vi "Get Control Data.vi"(6 "offset":i32, 8 "error in (no error)":errorcluster, 11 "bitfile xml in":string) -> (0 "error out":errorcluster, 2 "Controls":T1[](array[typedef]), 3 "Indicators":T1[](array[typedef]), 4 "offset past EndTag":i32)   [LabVIEW 2010, in "FPGA Bitfile Utility.lvlib"]
uses:
  <userlib>/_FPGA Interface Advanced Tools/FPGA Bitfile Utility/FPGA Bitfile Utility.lvlib
  <userlib>/_FPGA Interface Advanced Tools/FPGA Bitfile Utility/TypeDefs/Control_Indicator Info.ctl
  <vilib>/rvi/DataTransferAndStorage/Container/Common/niFpgaDataTypeControl.ctl
  <vilib>/rvi/Utilities/XML/nirviXML_GetValue.vi
  <vilib>/rvi/Utilities/XML/nirviXML_GetValue_String.vi
  <vilib>/rvi/Bitfile/niFpgaReadBitfileXml_VIRegisterMap.vi
  <vilib>/rvi/Utilities/XML/nirviXML_GetValue_U32.vi
  <vilib>/Utility/VariantDataType/VariantType.lvlib
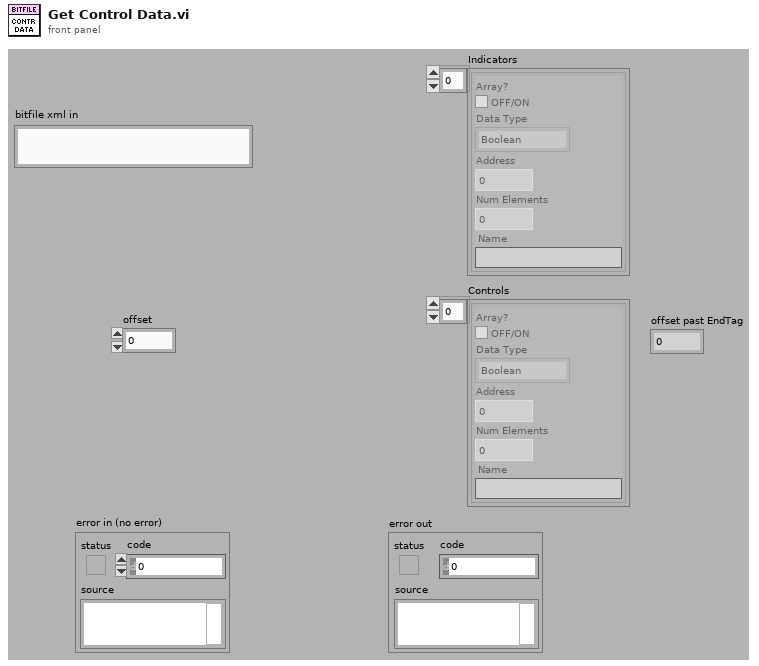
[diagram p1: front panel]
types:
  T1 = typedef "FPGA Bitfile Utility.lvlib/Control_Indicator Info.ctl" = cluster{"Array?":bool, "Data Type":T2, "Address":u32, "Num Elements":u32, "Name":string}
  T2 = typedef "niFpgaDataTypeControl.ctl" = enum32{"Boolean", "I8", "I16", "I32", "I64", "U8", "U16", "U32", "U64", "FXP", "CustomControl"}
  T3 = typedef "nirviControlStructure.ctl" = cluster{"Name":string, "Hidden":bool, "Indicator":bool, "Flattened Type":string, "Grouping":cluster{"Grouped":bool, "Member Names":string[], "Member IDs":u32[]}, "Address":u32, "Size":u32, "Class":u32, "Internal":bool, "Typedef":T4, "ID":u32, "Bidirectional":bool, "Synchronous":bool, "Mechanical Action":T5, "Sub Controls":T6[], "Access May Timeout":bool, "Register Node":bool}
  T4 = typedef "nirviTypdefDescription.ctl" = cluster{"Typedef":bool, "Path":path}
  T5 = typedef "nirviMechanicalAction.ctl" = enum8{"Switch When Pressed", "Switch When Released", "Switch Until Released", "Latch When Pressed", "Latch When Released", "Latch Until Released"}
  T6 = typedef "nirviSubControlStructure.ctl" = cluster{"Name":string, "flattened Type":string, "Cluster Information":T7, "Typedef":T4}
  T7 = typedef "nirviClusterElementControl.ctl" = cluster{"Name Hierarchy":string[], "Item Order":u32[]}
  T8 = typedef "VariantType.lvlib/Type.ctl" = enum8{"Invalid Type", "Void", "I8", "I16", "I32", "I64", "U8", "U16", "U32", "U64", "Single Float", "Double Float", "Extended Float", "Single Complex", "Double Complex", "Extended Complex", "Enum U8", "Enum U16", "Enum U32", "Enum U64", "Single Float With Unit", "Double Float With Unit", "Extended Float With Unit", "Single Complex with Unit", "Double Complex with Unit", "Extended Complex with Unit", "Boolean", "String", "Path", "Picture", "Tag", "Array", "Cluster", "Variant", "LV Variant", "Waveform", "Timestamp", "Digital Waveform", "Digital Data", "ExpressData", "Refnum", "External Data", "VI", "Poly VI", "LabVIEW Class Instance", "Fixed Point"}
  T9 = typedef "VariantType.lvlib/MemoryInfo.ctl" = cluster{"Type":T10, "Size":u32}
  T10 = typedef "VariantType.lvlib/MemoryType.ctl" = enum16{"Variable", "Fixed", "Bounded"}
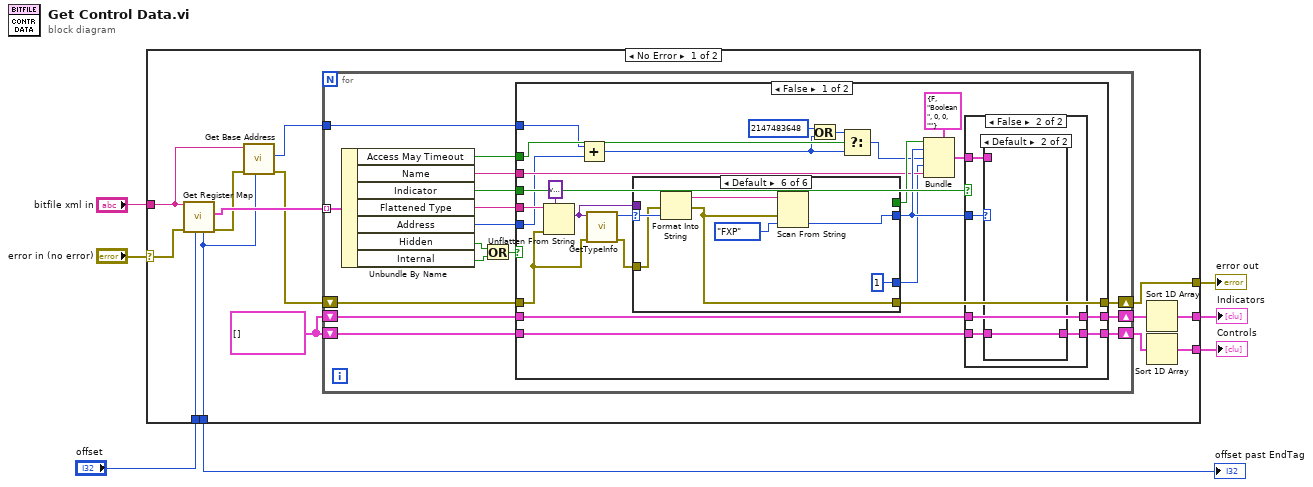
[diagram p0: block diagram]
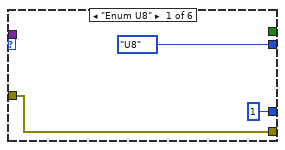
[diagram p2: hidden frame]
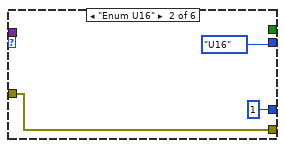
[diagram p3: hidden frame]
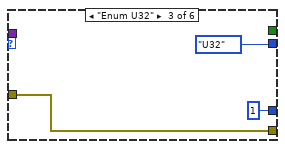
[diagram p4: hidden frame]
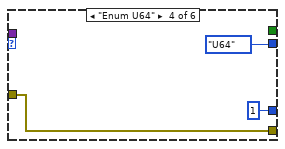
[diagram p5: hidden frame]
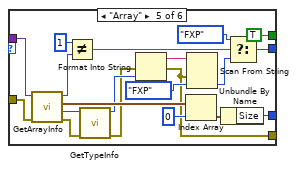
[diagram p6: hidden frame]
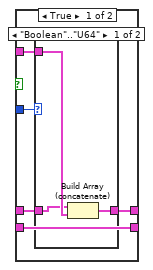
[diagram p7: hidden frame]
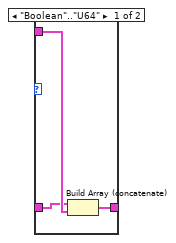
[diagram p9: hidden frame]
diagram:
  n1 = case shown="No Error" "error in (no error)" {
    selector: "error in (no error)" -> [w15 w124]
    tunnel: "bitfile xml in" -> [w12 _]
    tunnel: [w18 _] -> w6
    tunnel: [w17 _] -> w5
    tunnel: [w16 w124] -> w4
    tunnel: "offset" -> [w13 w123]
    tunnel: [w10 w123] -> w1
    frame No Error {
      w21 = T1[] []
      n2 = call <userlib>:"Get Register Map.vi"("offset"=w13, "error in (no error)"=w15, "bitfile xml in"=w12) -> ("error out"=w11:errorcluster, "register map"=w14:T3[], "offset past EndTag"=w10:i32)  [unwired: 6 in]
      n3 = call <userlib>:"Get Base Address.vi"("offset"=w10, "error in (no error)"=w11, "bitfile xml in"=w12) -> ("error out"=w8:errorcluster, "value"=w9:u32)  [unwired: 7 in]
      n4 = for {
        tunnel: w14 -> [w37] mode=indexing
        shift-right: [w24] -> w16
        shift-left: w8 -> [w29]
        shift-right: [w28] -> w20
        shift-left: w21 -> [w27]
        shift-right: [w26] -> w19
        shift-left: w21 -> [w25]
        tunnel: w9 -> [w22]
        n5 = Unbundle By Name(w37) -> ("Access May Timeout"=w23:bool, "Name"=w33:string, "Indicator"=w32:bool, "Flattened Type"=w31:string, "Address"=w30:u32, "Hidden"=w36:bool, "Internal"=w35:bool)
        n6 = Or(x=w36, y=w35) -> (x .or. y?=w34:bool)
        n7 = case shown="False" w34 {
          tunnel: w33 -> [w46 _]
          tunnel: w32 -> [w59 _]
          tunnel: w31 -> [w62 _]
          tunnel: w30 -> [w42 _]
          tunnel: w29 -> [w60 w120]
          tunnel: [w56 w122] -> w28
          tunnel: w27 -> [w55 w122]
          tunnel: [w54 w121] -> w26
          tunnel: w25 -> [w53 w121]
          tunnel: [w49 w120] -> w24
          tunnel: w23 -> [w41 _]
          tunnel: w22 -> [w38 _]
          frame False {
            n8 = Unflatten From String(type=variant ("variant"), binary string=w62, error in (no error)=w60) -> (value=w52:variant)  [unwired: 2 in, 2 out]
            n9 = Add(x=w38, y=w42) -> (x+y=w39:u32)
            n10 = call <vilib>:"GetTypeInfo.vi"("error in (no error)"=w60, "Variant"=w52) -> ("error out"=w51:errorcluster, "Type Enum"=w57:T8)  [unwired: 5 in, 3 out]
            n11 = case shown="Default" w57 {
              selector: w57 -> [_ _ _ _ _ w100]
              tunnel: [niFpgaDataTypeControl."U8" ("Data Type") niFpgaDataTypeControl."U16" ("Data Type") niFpgaDataTypeControl."U32" ("Data Type") niFpgaDataTypeControl."U64" ("Data Type") w86 w96] -> w47
              tunnel: w52 -> [_ _ _ _ w94 _]
              tunnel: w51 -> [w65 w68 w71 w74 w93 w99]
              tunnel: [_ _ _ _ TRUE ("Indicator") _] -> w48
              tunnel: [w65 w68 w71 w74 w75 w95] -> w49
              tunnel: [u32 1 ("Size") u32 1 ("Size") u32 1 ("Size") u32 1 ("Size") w82 u32 1 ("Size")] -> w45
              frame "Enum U8" {
              }
              frame "Enum U16" {
              }
              frame "Enum U32" {
              }
              frame "Enum U64" {
              }
              frame "Array" {
                n12 = call <vilib>:"GetArrayInfo.vi"("error in (no error)"=w93, "Variant"=w94) -> ("error out"=w88:errorcluster, "ArrayElement"=w87:variant, "Array Lengths"=w85:T9[], "NDims"=w91:i32)  [unwired: 6 in]
                n13 = Not Equal?(x=1, y=w91) -> (x != y?=w89:bool)
                n14 = call <vilib>:"GetTypeInfo.vi"("error in (no error)"=w88, "Variant"=w87) -> ("error out"=w76:errorcluster, "Type Enum"=w77:T8)  [unwired: 5 in, 3 out]
                n15 = Format Into String(error in=w76, w77) -> (resulting string=w80:string, error out=w75:errorcluster)  [unwired: 2 in]
                n16 = Index Array(array=w85, index=0) -> (element=w83:T9)
                n17 = Scan From String(input string=w80, error in=w75, default 1=niFpgaDataTypeControl."FXP" ("Data Type")) -> (output 1=w78:T2)  [unwired: 2 in, 3 out]
                n18 = Unbundle By Name(w83) -> ("Size"=w82:u32)
                n19 = Select(t=niFpgaDataTypeControl."FXP" ("Data Type"), s=w89, f=w78) -> (s? t:f=w86:T2)
              }
              frame Default {
                n20 = Format Into String(error in=w99, w100) -> (resulting string=w98:string, error out=w95:errorcluster)  [unwired: 2 in]
                n21 = Scan From String(input string=w98, error in=w95, default 1=niFpgaDataTypeControl."FXP" ("Data Type")) -> (output 1=w96:T2)  [unwired: 2 in, 3 out]
              }
            }
            n22 = Or(x=u32 2147483648 ("Address"), y=w39) -> (x .or. y?=w43:u32)
            n23 = Select(t=w43, s=w41, f=w39) -> (s? t:f=w40:u32)
            n24 = Bundle(cluster=T1 {"Array?"=FALSE, "Data Type"=enum."Boolean", "Address"=0, "Num Elements"=0, "Name"=""}, "Array?"=w48, "Data Type"=w47, "Address"=w40, "Num Elements"=w45, "Name"=w46) -> (w58:T1)
            n25 = case shown="False" w59 {
              tunnel: w47 -> [w106 w115]
              tunnel: w58 -> [w105 w114]
              tunnel: [w104 w111] -> w56
              tunnel: w55 -> [w103 w111]
              tunnel: [w102 w113] -> w54
              tunnel: w53 -> [w102 w112]
              frame True {
                n26 = case shown="\"Boolean\"..\"U64\"" w106 {
                  tunnel: w105 -> [w109 _]
                  tunnel: [w108 w110] -> w104
                  tunnel: w103 -> [w107 w110]
                  frame "Boolean".."U64" {
                    n27 = Build Array (concatenate)(w107, w109) -> (w108:T1[])
                  }
                  frame Default {
                  }
                }
              }
              frame False {
                n28 = case shown="Default" w115 {
                  tunnel: w114 -> [w118 _]
                  tunnel: [w117 w119] -> w113
                  tunnel: w112 -> [w116 w119]
                  frame "Boolean".."U64" {
                    n29 = Build Array (concatenate)(w116, w118) -> (w117:T1[])
                  }
                  frame Default {
                  }
                }
              }
            }
          }
          frame True {
          }
        }
      }
      n30 = Sort 1D Array(array=w20) -> (sorted array=w18:T1[])
      n31 = Sort 1D Array(array=w19) -> (sorted array=w17:T1[])
    }
    frame Error {
    }
  }
  "Indicators" <- w6
  "Controls" <- w5
  "error out" <- w4
  "offset past EndTag" <- w1
